vi "target_trajectory.vi"(0 "start_test":bool) -> (1 "start":bool, 2 "target_x":dbl, 3 "target_y":dbl, 4 "done":bool)   [LabVIEW 2019]
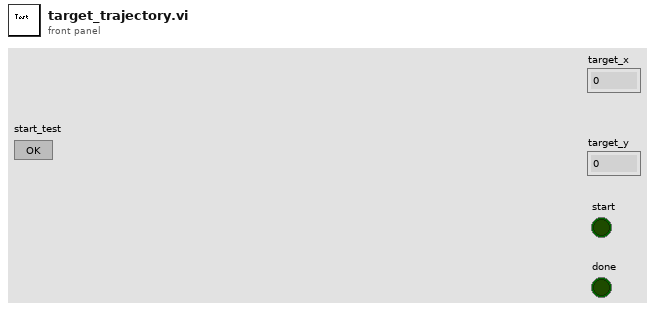
[diagram p1: front panel]
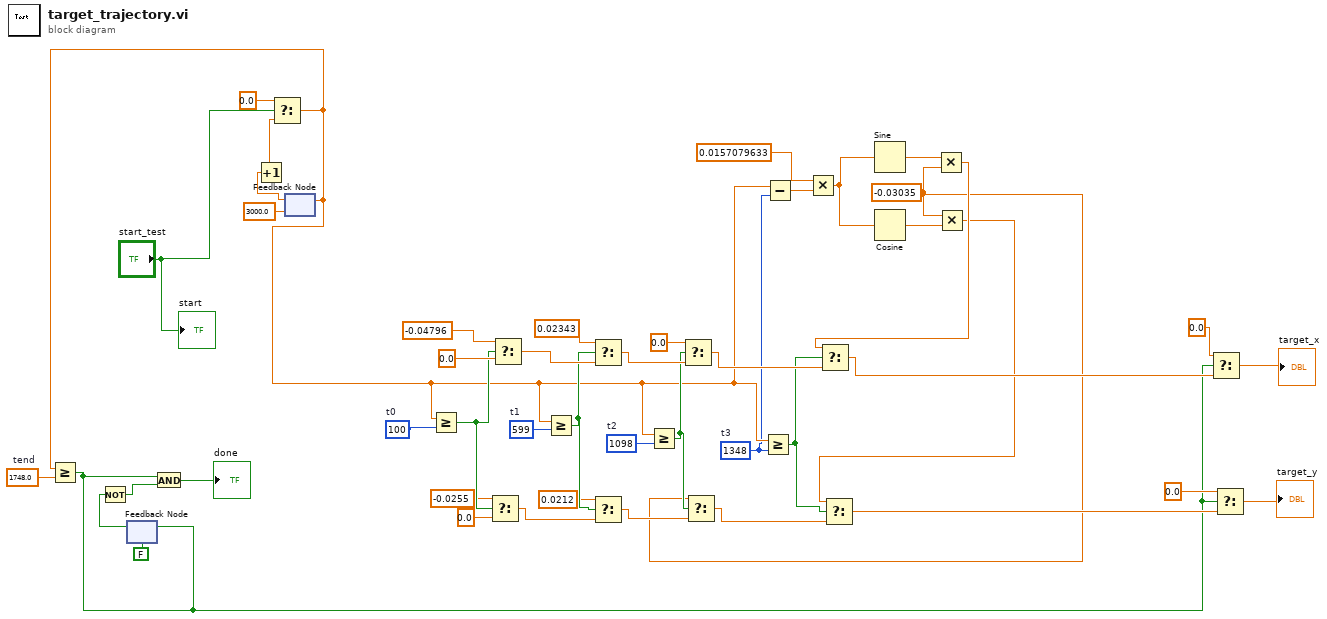
[diagram p0: block diagram]
diagram:
  w6 = -0.03035
  w15 = 1348  # t3
  w31 = 1098  # t2
  w34 = 599  # t1
  w41 = 100  # t0
  w44 = 1748.0  # tend
  n1 = feedback #1(FALSE) -> (w4:bool)
  n2 = Not(x=w4) -> (.not. x?=w3:bool)
  n3 = feedback #2(3000.0 ("t")) -> (w43:dbl)
  n4 = Increment(x=w43) -> (x+1=w42:dbl)
  n5 = Select(t=0.0, s="start_test", f=w42) -> (s? t:f=w16:dbl)
  n6 = Greater Or Equal?(x=w16, y=w44) -> (x >= y?=w2:bool)
  n7 = feedback-in #1(w2) -> ()
  n8 = And(x=w2, y=w3) -> (x .and. y?=→"done":bool)
  n9 = feedback-in #2(w16) -> ()
  n10 = Greater Or Equal?(x=w16, y=w41) -> (x >= y?=w26:bool)
  n11 = Select(t=-0.0255, s=w26, f=0.0) -> (s? t:f=w23:dbl)
  n12 = Select(t=-0.04796, s=w26, f=0.0) -> (s? t:f=w33:dbl)
  n13 = Greater Or Equal?(x=w16, y=w34) -> (x >= y?=w27:bool)
  n14 = Select(t=0.02343, s=w27, f=w33) -> (s? t:f=w30:dbl)
  n15 = Select(t=0.0212, s=w27, f=w23) -> (s? t:f=w22:dbl)
  n16 = Greater Or Equal?(x=w16, y=w31) -> (x >= y?=w28:bool)
  n17 = Select(t=0.0, s=w28, f=w30) -> (s? t:f=w20:dbl)
  n18 = Select(t=w6, s=w28, f=w22) -> (s? t:f=w19:dbl)
  n19 = Greater Or Equal?(x=w16, y=w15) -> (x >= y?=w8:bool)
  n20 = Subtract(x=w16, y=w15) -> (x-y=w14:dbl)
  n21 = Multiply(x=0.0157079633, y=w14) -> (x*y=w13:dbl)
  n22 = Sine(x=w13) -> (sin(x)=w12:dbl)
  n23 = Cosine(x=w13) -> (cos(x)=w11:dbl)
  n24 = Multiply(x=w12, y=w6) -> (x*y=w10:dbl)
  n25 = Select(t=w10, s=w8, f=w20) -> (s? t:f=w17:dbl)
  n26 = Multiply(x=w6, y=w11) -> (x*y=w9:dbl)
  n27 = Select(t=w9, s=w8, f=w19) -> (s? t:f=w18:dbl)
  n28 = Select(t=0.0, s=w2, f=w17) -> (s? t:f=→"target_x":dbl)
  n29 = Select(t=0.0, s=w2, f=w18) -> (s? t:f=→"target_y":dbl)
  "start" <- "start_test"
